vi "SetAppMetadataProperty.vi"(8 "No Error":errorcluster, 9 "Remove Property (F)":bool, 10 "Value (\"\")":string, 11 "Name":T1) -> (0 "error out":errorcluster)   [LabVIEW 2026, in "SDL3.lvlib" / "Init.lvlib"]
doc: "<B>Summary</B>\nSpecify metadata about your app through a set of properties.\n\n<B>Remarks</B>\nYou can optionally provide metadata about your app to SDL. This is not required, but strongly encouraged.\n\nThere are several locations where SDL can make use of metadata (an \"About\" box in the macOS menu bar, the name of the app can be shown on some audio mixers, etc). Any piece of metadata can be left out, if a specific detail doesn't make sense for the app.\n\nThis function should be called as early as possible, before <B>SDL_Init</B>. Multiple calls to this function are allowed, but various state might not change once it has been set up with a previous call to this function.\n\nOnce set, this metadata can be read using <B>SDL_GetMetadataProperty()</B>.\n\nThese are the supported properties:\n\n- <B>SDL_PROP_APP_METADATA_NAME_STRING</B>: The human-readable name of the application, like \"My Game 2: Bad Guy's Revenge!\". This will show up anywhere the OS shows the name of the application separately from window titles, such as volume control applets, etc. This defaults to \"SDL Application\".\n- <B>SDL_PROP_APP_METADATA_VERSION_STRING</B>: The version of the app that is running; there are no rules on format, so \"1.0.3beta2\" and \"April 22nd, 2024\" and a git hash are all valid options. This has no default.\n- <B>SDL_PROP_APP_METADATA_IDENTIFIER_STRING</B>: A unique string that identifies this app. This must be in reverse-domain format, like \"com.example.mygame2\". This string is used by desktop compositors to identify and group windows together, as well as match applications with associated desktop settings and icons. If you plan to package your application in a container such as Flatpak, the app ID should match the name of your Flatpak container as well. This has no default.\n- <B>SDL_PROP_APP_METADATA_CREATOR_STRING</B>: The human-readable name of the creator/developer/maker of this app, like \"MojoWorkshop, LLC\"\nSDL_PROP_APP_METADATA_COPYRIGHT_STRING</B>: The human-readable copyright notice, like \"Copyright (c) 2024 MojoWorkshop, LLC\" or whatnot. Keep this to one line, don't paste a copy of a whole software license in here. This has no default.\n- <B>SDL_PROP_APP_METADATA_URL_STRING</B>: A URL to the app on the web. Maybe a product page, or a storefront, or even a GitHub repository, for user's further information This has no default.\n- <B>SDL_PROP_APP_METADATA_TYPE_STRING</B>: The type of application this is. Currently this string can be \"game\" for a video game, \"mediaplayer\" for a media player, or generically \"application\" if nothing else applies. Future versions of SDL might add new types. This defaults to \"application\"."
uses:
  Init.lvlib
  MetadataPropertyName--combobox.ctl
  <vilib>/Utility/error.llb/Error Cluster From Error Code.vi
  Error/Error.lvlib
  Lib/SDL3.dll
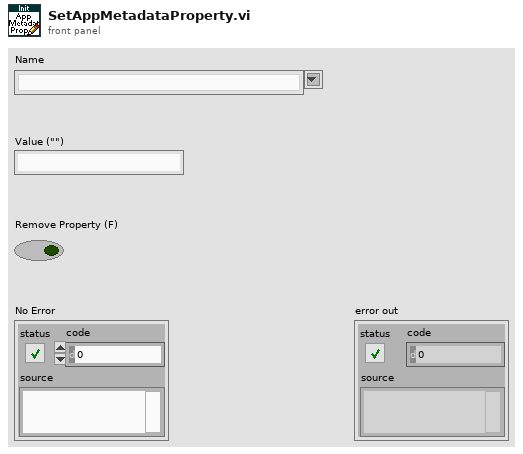
[diagram p1: front panel]
types:
  T1 = typedef "SDL3.lvlib/Init.lvlib/MetadataPropertyName--combobox.ctl" = string
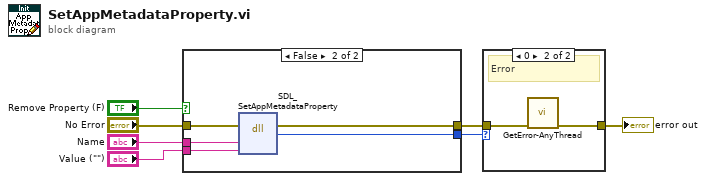
[diagram p0: block diagram]
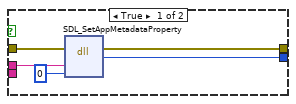
[diagram p2: hidden frame]
diagram:
  n1 = case shown="False" "Remove Property (F)" {
    tunnel: "No Error" -> [w12 w17]
    tunnel: [w11 w16] -> w5
    tunnel: [w10 w15] -> w4
    tunnel: "Name" -> [w9 w14]
    tunnel: "Value (\"\")" -> [_ w13]
    frame True {
      n2 = dll-call lib="C:/Users/saukko/Dev/LV-SDL3/Sources/SDL3/Lib/SDL3.*" fn="SDL_SetAppMetadataProperty"(error in=w12, "name"=w9, "value"=i64 0) -> (error out=w10:errorcluster, "return type"=w11:i32)  [unwired: 4 in, 1 out]
    }
    frame False {
      n3 = dll-call lib="C:/Users/saukko/Dev/LV-SDL3/Sources/SDL3/Lib/SDL3.*" fn="SDL_SetAppMetadataProperty"(error in=w17, "name"=w14, "value"=w13) -> (error out=w15:errorcluster, "return type"=w16:i32)  [unwired: 4 in, 1 out]
    }
  }
  n4 = case shown="0" w5 {
    tunnel: w4 -> [w18 w20]
    tunnel: [w18 w19] -> w6
    frame Default {
      # "Ok"
    }
    frame 0 {
      # "Error"
      n5 = call "GetError-AnyThread.vi"("No Error"=w20) -> ("Error Out"=w19:errorcluster)  [unwired: 10 in]
    }
  }
  "error out" <- w6
